vi "Set Tx Generic Properties.vi"(8 "error in":errorcluster, 10 "session_tx_generic":T1={"tx_generic_setup"={"QueueSizeIn"=0, "Count"=12, "StartMode"=1}, "Frame Headers"=[]} {"Frame Headers"."Frame header"."SequenceNumberOffset" items=["FDX_TX_FRAME_SEQ_OFFS_AUTO"=65535]; "Frame Headers"."Frame header"."SequenceNumberInit" items=["FDX_TX_FRAME_SEQ_INIT_AUTO"=65535, "FDX_TX_FRAME_SEQ_OFF"=65533]; "Frame Headers"."Frame header"."PhysErrorInjection" items=["FDX_TX_FRAME_ERR_OFF", "FDX_TX_FRAME_ERR_CRC", "FDX_TX_FRAME_ERR_ALI", "FDX_TX_FRAME_ERR_PRE", "FDX_TX_FRAME_ERR_PHY"]; "Frame Headers"."Frame header"."PayloadGenerationMode" items=["FDX_TX_FRAME_PGM_USER", "FDX_TX_FRAME_PGM_IP_PART", "FDX_TX_FRAME_PGM_IP_PART_TT", "FDX_TX_FRAME_PGM_IP_FULL", "FDX_TX_FRAME_PGM_IP_FULL_TT"]; "Frame Headers"."Frame header"."PayloadBufferMode" items=["FDX_TX_FRAME_PBM_STD", "FDX_TX_FRAME_PBM_MAC", "FDX_TX_FRAME_PBM_UDP", "FDX_TX_FRAME_PBM_FULL"]; "Frame Headers"."Frame header"."NetSelect" items=["FDX_TX_FRAME_DLY_A"=0, "FDX_TX_FRAME_DLY_B"=1, "FDX_TX_FRAME_BOTH "=3, "FDX_TX_FRAME_ONLY_A"=4, "FDX_TX_FRAME_ONLY_B "=5]; "Frame Headers"."Frame header"."FrameStartMode" items=["FDX_TX_FRAME_START_IFG", "FDX_TX_FRAME_START_PGWT", "FDX_TX_FRAME_START_TRG", "FDX_TX_FRAME_START_TRG_D"]; "tx_generic_setup"."StartMode" items=["FDX_STOP", "FDX_START", "FDX_START_TRG", "FDX_START_TIME"]}, 11 "custom device ref in":T9 format="%.0x") -> (0 "error out":errorcluster, 3 "custom device ref out":T9 format="%.0x")   [LabVIEW 2020, in "AIM ARINC 664 Scripting.lvlib"]
uses:
  AIM ARINC 664 Scripting.lvlib
  <vilib>/NI VeriStand/Custom Device API/Custom Device API.lvlib
  <vilib>/NI VeriStand/Custom Device API/Set Item Property (U32).vi
  Constants.vi
  <vilib>/NI VeriStand/Custom Device API/Custom Device Item Ref.ctl
  Import/_typedefs/session_tx_generic.ctl
  Import/AIM ARINC 664 Import.lvlib
  Import/_typedefs/tx_generic_setup.ctl
  Import/_typedefs/frame_tx_generic_seqNumberInit.ctl
  Import/_typedefs/frame_tx_generic_seqNumberOffset.ctl
  Import/_typedefs/frame_tx_generic.ctl
  Import/_typedefs/frame_parameter_definition.ctl
  Import/_typedefs/frame_parameter.ctl
  Shared/Encoding (Arinc664).ctl
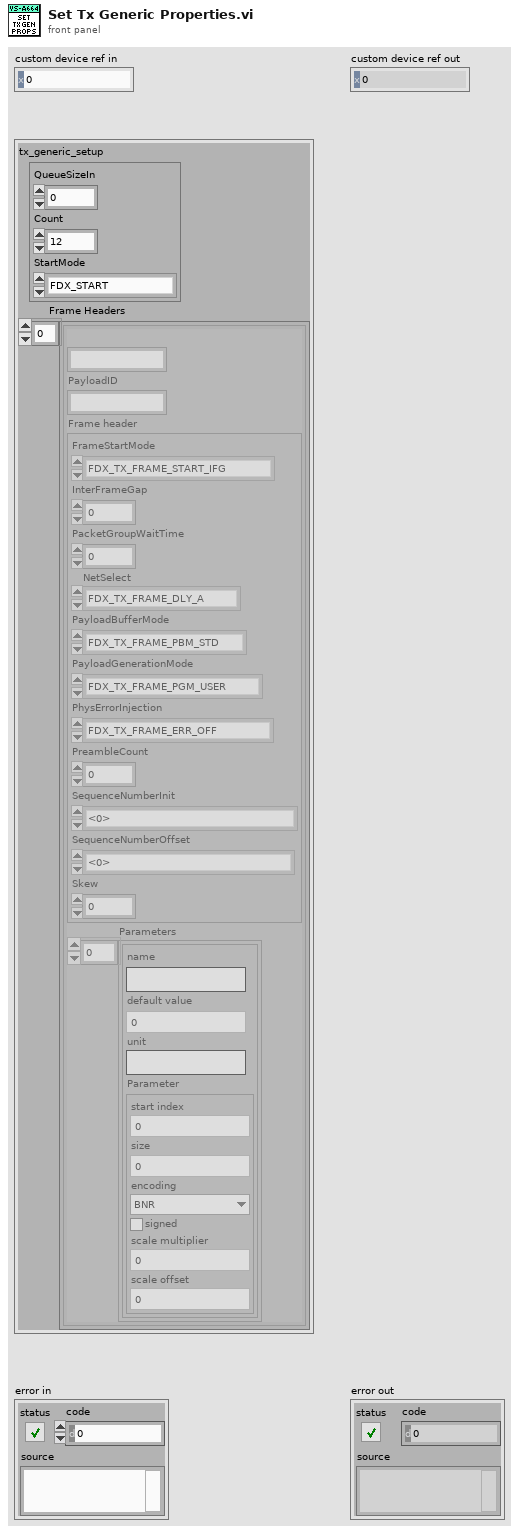
[diagram p1: front panel]
types:
  T1 = typedef "AIM ARINC 664 Import.lvlib/session_tx_generic.ctl" = cluster{"tx_generic_setup":T2, "Frame Headers":T3[]}
  T2 = typedef "AIM ARINC 664 Import.lvlib/tx_generic_setup.ctl" = cluster{"QueueSizeIn":u32, "Count":i32, "StartMode":i32}
  T3 = typedef "AIM ARINC 664 Import.lvlib/frame_tx_generic.ctl" = cluster{"FrameID":string, "PayloadID":string, "Frame header":cluster{"FrameStartMode":i32, "InterFrameGap":i32, "PacketGroupWaitTime":i32, "NetSelect":u32, "PayloadBufferMode":i32, "PayloadGenerationMode":i32, "PhysErrorInjection":i32, "PreambleCount":i32, "SequenceNumberInit":T4, "SequenceNumberOffset":T5, "Skew":i32}, "Parameters":T6[]}
  T4 = typedef "AIM ARINC 664 Import.lvlib/frame_tx_generic_seqNumberInit.ctl" = i32
  T5 = typedef "AIM ARINC 664 Import.lvlib/frame_tx_generic_seqNumberOffset.ctl" = i32
  T6 = typedef "AIM ARINC 664 Import.lvlib/frame_parameter.ctl" = cluster{"name":string, "default value":dbl, "unit":string, "Parameter":T7}
  T7 = typedef "AIM ARINC 664 Import.lvlib/frame_parameter_definition.ctl" = cluster{"start index":i32, "size":i32, "encoding":T8, "signed":bool, "scale multiplier":dbl, "scale offset":dbl}
  T8 = typedef "Encoding (Arinc664).ctl" = enum16{"BNR", "BCD", "Discrete"}
  T9 = typedef "Custom Device API.lvlib/Custom Device Item Ref.ctl" = u64
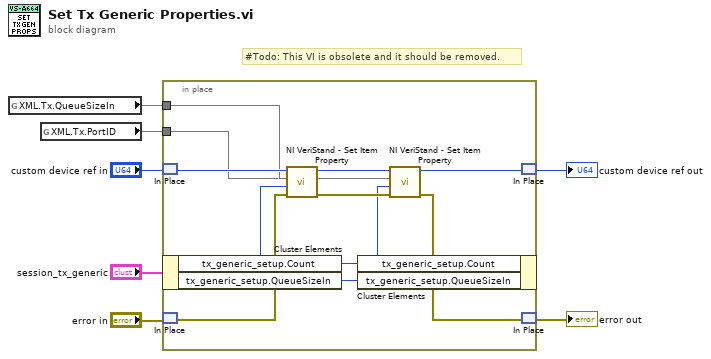
[diagram p0: block diagram]
diagram:
  # "#Todo: This VI is obsolete and it should be removed."
  n1 = global read "Constants.vi" "XML.Tx.QueueSizeIn"() -> (w3)
  n2 = global read "Constants.vi" "XML.Tx.PortID"() -> (w2)
  n3 = in-place {
    in-place-border: w3 -> [w9]
    in-place-border: w2 -> [w8]
    n4 = in-place-match #1("custom device ref in") -> (w13:T9)
    n5 = in-place-cluster #2("session_tx_generic") -> ("tx_generic_setup.Count"=w15:i32, "tx_generic_setup.QueueSizeIn"=w11:u32)
    n6 = in-place-match #3("error in") -> (w17:errorcluster)
    n7 = call-poly <vilib>:"NI VeriStand - Set Item Property.vi"("error in (no error)"=w17, "Value"=w15, "Property Name"=w8, "Item Ref in"=w13) -> ("error out"=w14:errorcluster, "Item Ref out"=w12:T9)  [unwired: 5 in, 1 out]
    n8 = in-place-cluster #2("tx_generic_setup.Count"=w15, "tx_generic_setup.QueueSizeIn"=w11) -> ()  [unwired: 1 out]
    n9 = call-poly <vilib>:"NI VeriStand - Set Item Property.vi"("error in (no error)"=w14, "Value"=w11, "Property Name"=w9, "Item Ref in"=w12) -> ("error out"=w16:errorcluster, "Item Ref out"=w10:T9)  [unwired: 5 in, 1 out]
    n10 = in-place-match #1(w10) -> (→"custom device ref out":T9)
    n11 = in-place-match #3(w16) -> (→"error out":errorcluster)
  }
